vi "Dispense FN - ON - State Status (SubVI).vi"(0 "Values IN":T1 {"Drain Time (s)" format="%.2f"; "Drain Rate (g/sec)" format="%.2f"}, 5 "Reverse/Purge Time (s)":dbl, 7 "Min Spray Complete?":bool, 8 "Spray Count":i32, 9 "Measure Delay Complete?":bool, 11 "Max Spray Complete?":bool, 13 "Reset?":bool) -> (14 "Values OUT":T1, 15 "Dispense Timeout?":bool, 16 "Purge Signal":bool, 17 "Complete":bool, 18 "Spray Signal":bool, 19 "OFF Signal":bool)   [LabVIEW 2011]
panel:
  out "Elapsed Time (s)":dbl
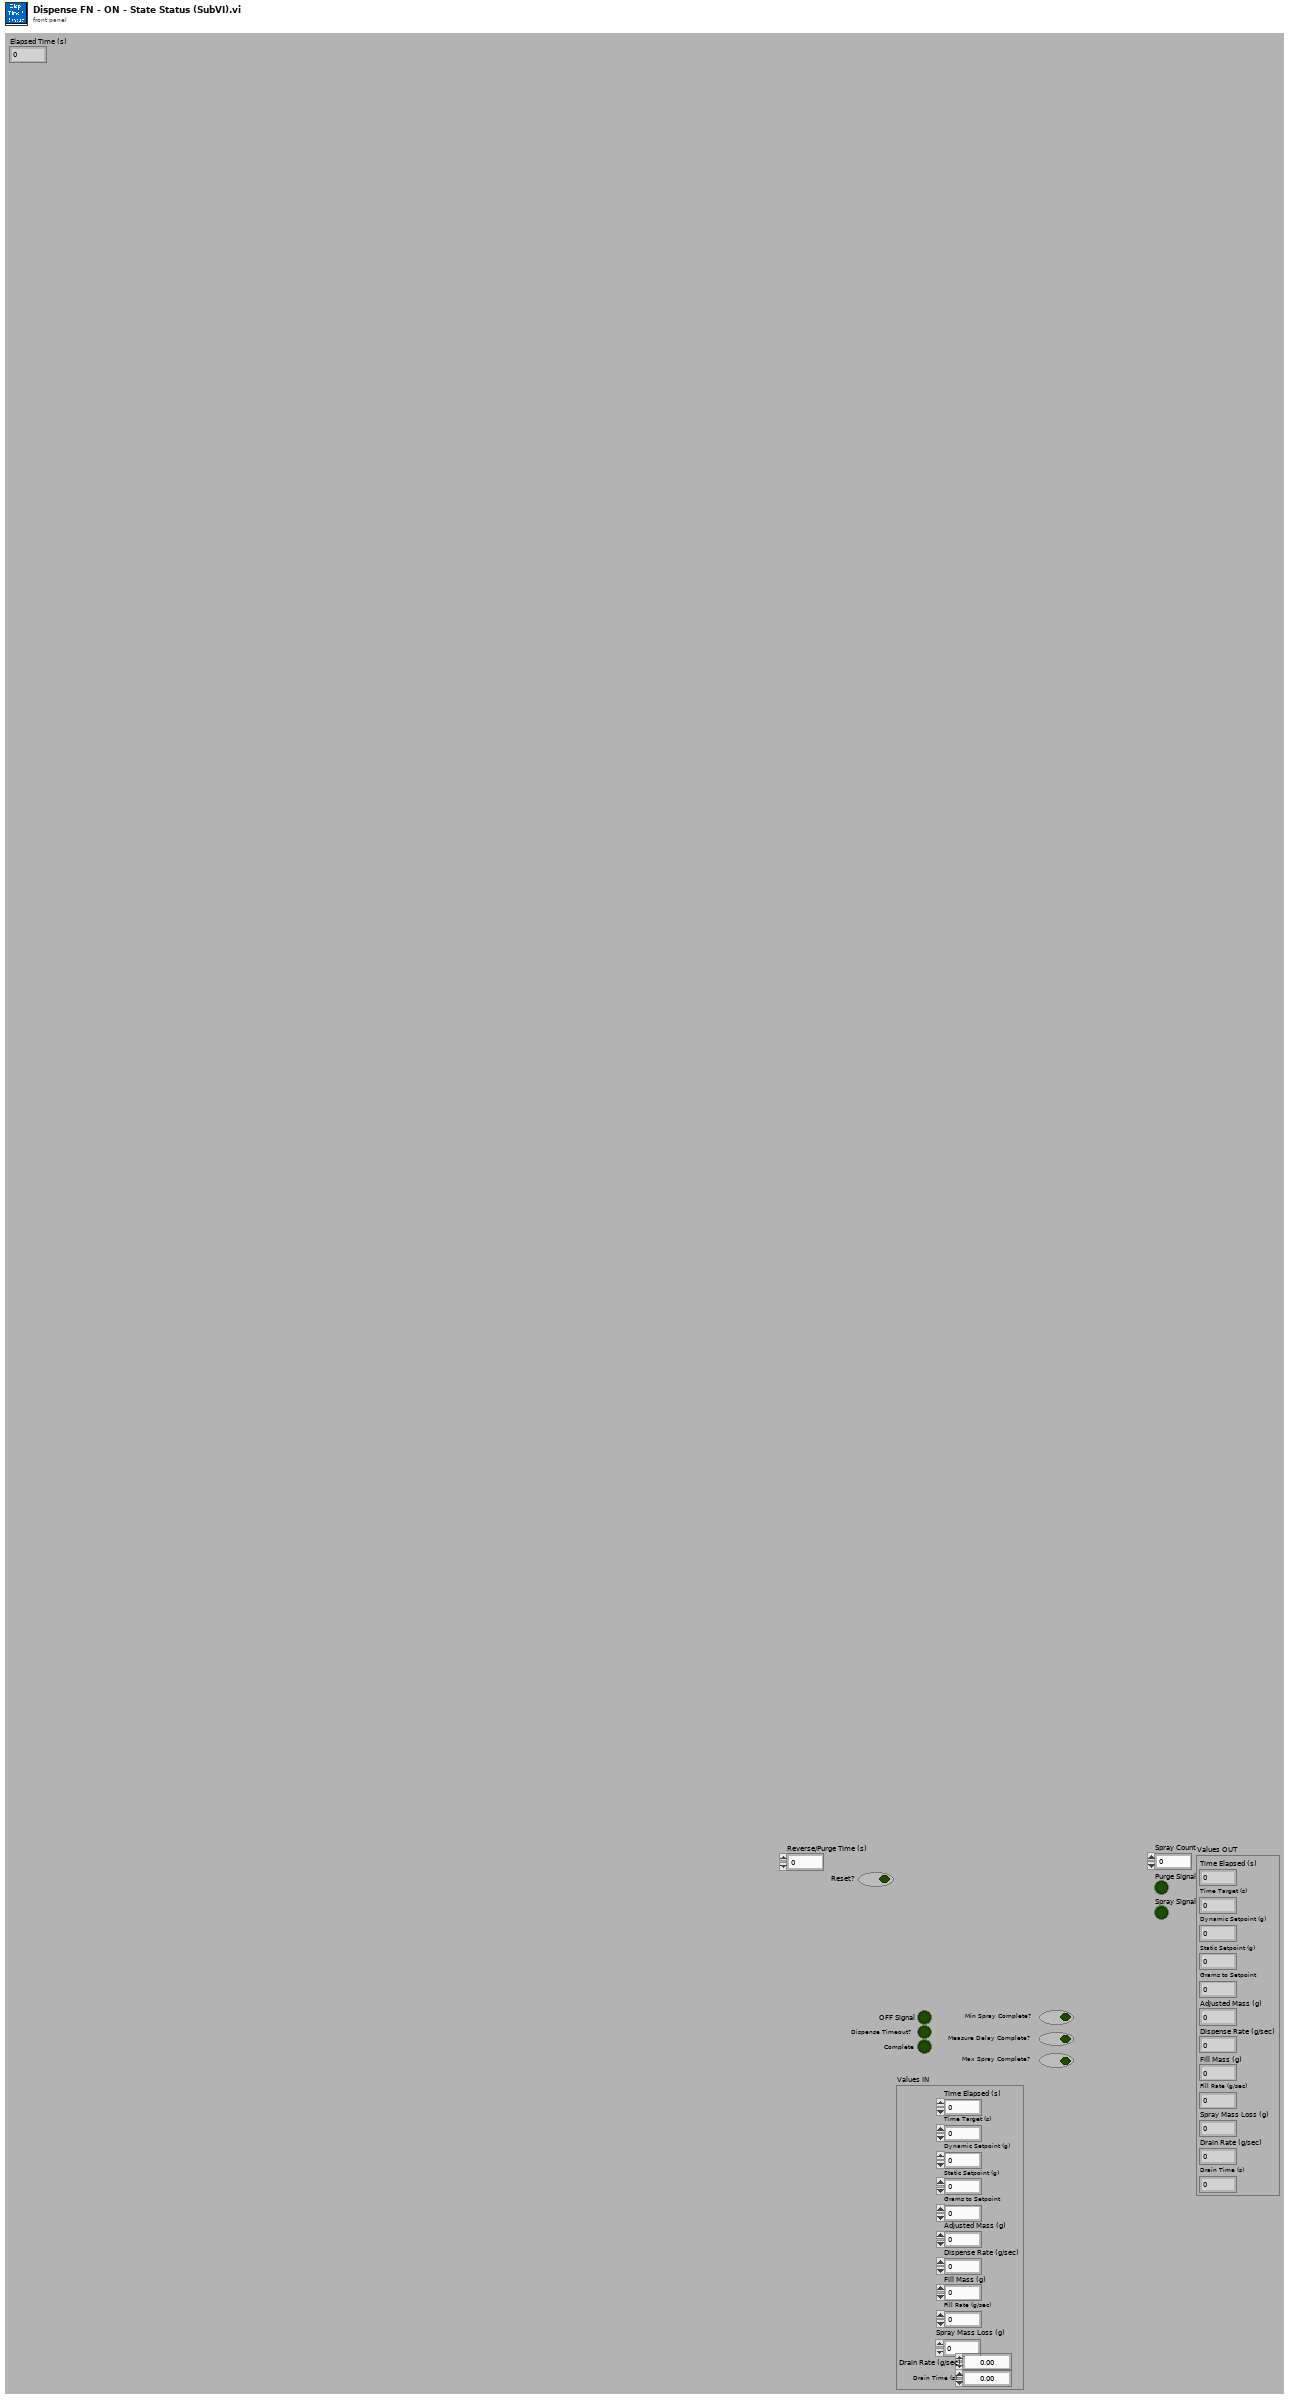
[diagram p1: front panel]
types:
  T1 = cluster{"Time Elapsed (s)":dbl, "Time Target (s)":dbl, "Dynamic Setpoint (g)":dbl, "Static Setpoint (g)":dbl, "Grams to Setpoint":dbl, "Adjusted Mass (g)":dbl, "Dispense Rate (g/sec)":dbl, "Fill Mass (g)":dbl, "Fill Rate (g/sec)":dbl, "Spray Mass Loss (g)":dbl, "Drain Rate (g/sec)":dbl, "Drain Time (s)":dbl}
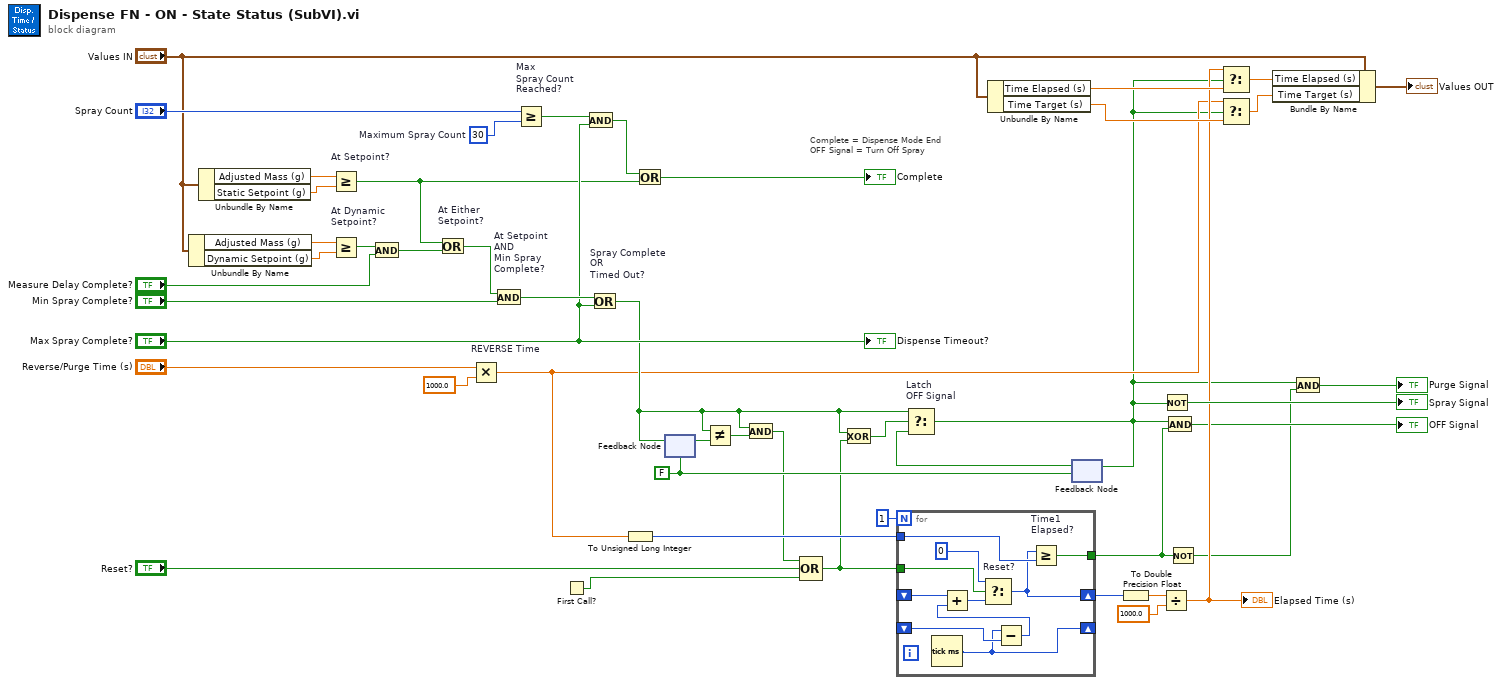
[diagram p0: block diagram]
diagram:
  w22 = FALSE
  w37 = 30  # Maximum Spray Count
  # "Complete = Dispense Mode End\nOFF Signal = Turn Off Spray"
  n1 = Unbundle By Name("Values IN") -> ("Adjusted Mass (g)"=w44:dbl, "Dynamic Setpoint (g)"=w45:dbl)
  n2 = Unbundle By Name("Values IN") -> ("Adjusted Mass (g)"=w47:dbl, "Static Setpoint (g)"=w46:dbl)
  n3 = Greater Or Equal? "At Setpoint?"(x=w47, y=w46) -> (x >= y?=w33:bool)
  n4 = Greater Or Equal? "At Dynamic\nSetpoint?"(x=w44, y=w45) -> (x >= y?=w48:bool)
  n5 = And(x=w48, y="Measure Delay Complete?") -> (x .and. y?=w41:bool)
  n6 = Or "At Either\nSetpoint?"(x=w33, y=w41) -> (x .or. y?=w40:bool)
  n7 = Multiply "REVERSE Time"(x="Reverse/Purge Time (s)", y=1000.0) -> (x*y=w6:dbl)
  n8 = And "At Setpoint\nAND\nMin Spray\nComplete?"(x=w40, y="Min Spray Complete?") -> (x .and. y?=w39:bool)
  n9 = Greater Or Equal? "Max\nSpray Count\nReached?"(x="Spray Count", y=w37) -> (x >= y?=w36:bool)
  n10 = First Call?() -> (First Call?: T/F=w21:bool)
  n11 = And(x=w36, y="Max Spray Complete?") -> (x .and. y?=w32:bool)
  n12 = Or "Spray Complete\nOR\nTimed Out?"(x=w39, y="Max Spray Complete?") -> (x .or. y?=w18:bool)
  n13 = To Unsigned Long Integer(number=w6) -> (unsigned 32bit integer=w26:u32)
  n14 = Or(x=w32, y=w33) -> (x .or. y?=→"Complete":bool)
  n15 = feedback #1(w22) -> (w31:bool)
  n16 = feedback-in #1(w18) -> ()
  n17 = Not Equal?(x=w18, y=w31) -> (x != y?=w30:bool)
  n18 = And(x=w18, y=w30) -> (x .and. y?=w20:bool)
  n19 = Compound Arithmetic op=OR(w20, "Reset?", w21) -> (w19:bool)
  n20 = Exclusive Or(1:w19, 2:w18) -> (0:w24:bool)
  n21 = for {
    N: 1 -> [_]
    shift-right: [w57] -> _
    shift-left: _ -> [w58]
    shift-right: [w50] -> w29
    shift-left: _ -> [w54]
    tunnel: w26 -> [w53]
    tunnel: [w52] -> w4
    tunnel: w19 -> [w49]
    n22 = Tick Count (ms)() -> (millisecond timer value=w57:u32)
    n23 = Subtract(x=w57, y=w58) -> (x-y=w51:u32)
    n24 = Add(x=w54, y=w51) -> (x+y=w56:u32)
    n25 = Select "Reset?"(t=u32 0, s=w49, f=w56) -> (s? t:f=w50:u32)
    n26 = Greater Or Equal? "Time1\nElapsed?"(x=w50, y=w53) -> (x >= y?=w52:bool)
  }
  n27 = Unbundle By Name("Values IN") -> ("Time Elapsed (s)"=w13:dbl, "Time Target (s)"=w11:dbl)
  n28 = feedback #2(w22) -> (w23:bool)
  n29 = Select "Latch\nOFF Signal"(t=w18, s=w24, f=w23) -> (s? t:f=w3:bool)
  n30 = feedback-in #2(w3) -> ()
  n31 = To Double Precision Float(number=w29) -> (double precision float=w28:dbl)
  n32 = Divide(x=w28, y=1000.0) -> (x/y=w7:dbl)
  "Elapsed Time (s)" <- w7
  n33 = Not(x=w3) -> (.not. x?=→"Spray Signal":bool)
  n34 = And(x=w3, y=w4) -> (x .and. y?=→"OFF Signal":bool)
  n35 = Not(x=w4) -> (.not. x?=w2:bool)
  n36 = Select(t=w7, s=w3, f=w13) -> (s? t:f=w12:dbl)
  n37 = Select(t=w6, s=w3, f=w11) -> (s? t:f=w10:dbl)
  n38 = Bundle By Name(cluster="Values IN", "Time Elapsed (s)"=w12, "Time Target (s)"=w10) -> (→"Values OUT":T1)
  n39 = And(x=w3, y=w2) -> (x .and. y?=→"Purge Signal":bool)
  "Dispense Timeout?" <- "Max Spray Complete?"
